vi "Graphics-Create Gradient.vi"(0 "intensity graph":refnum<vi>, 5 "Color 1":u32(colorbox)=16777216, 7 "Color 2":u32(colorbox)=16777215, 9 "Fraction":dbl, 11 "error in (no error)":errorcluster, 12 "Direction":T1(ring), 13 "Frame Color":u32(colorbox)=16777216) -> (15 "error out":errorcluster)   [LabVIEW 2020]
uses:
  Math VIs/LinSpace (x0-dx-npts).vi
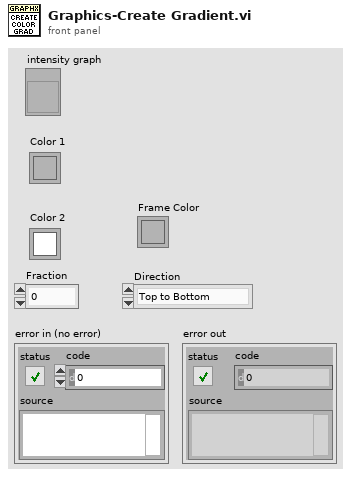
[diagram p1: front panel]
types:
  T1 = enum16{"Top to Bottom", "Bottom to Top", "Left to Right", "Right to Left"}
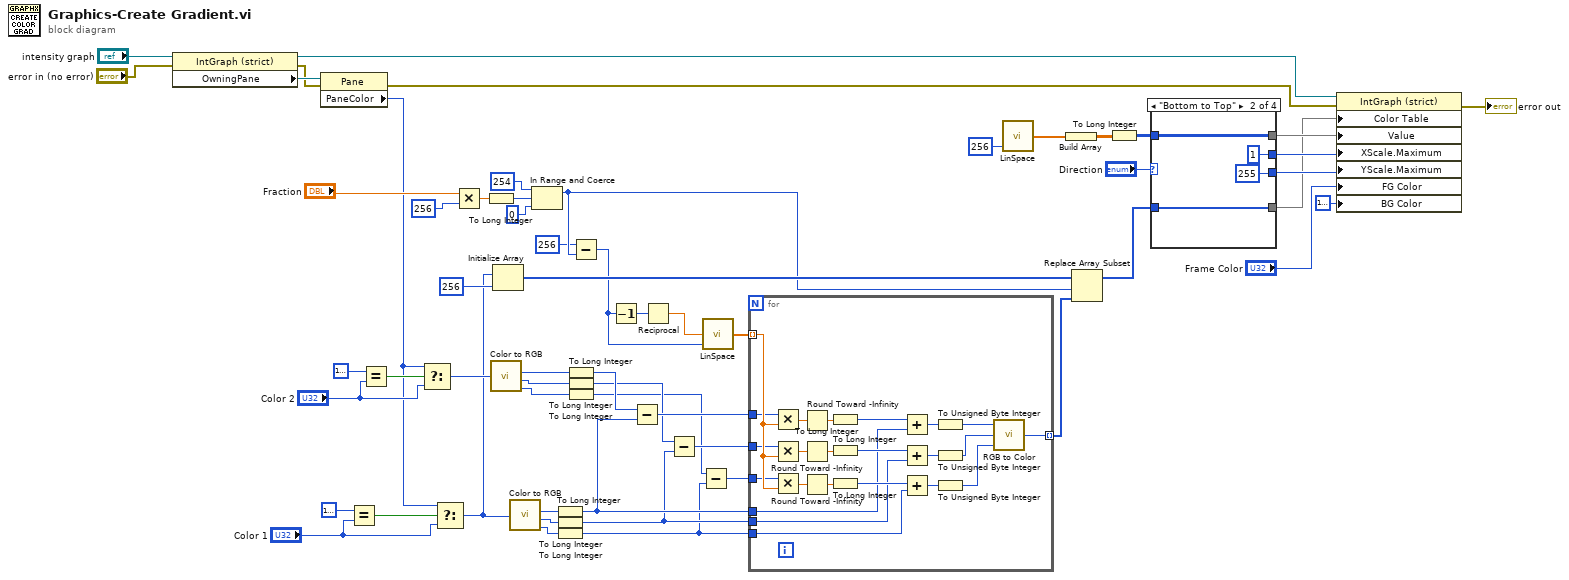
[diagram p0: block diagram]
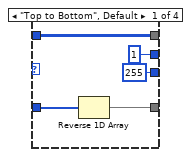
[diagram p2: hidden frame]
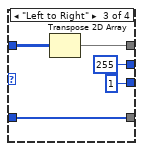
[diagram p3: hidden frame]
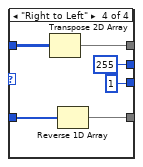
[diagram p4: hidden frame]
diagram:
  n1 = property class="IntGraph (strict)"(reference="intensity graph", error in="error in (no error)") -> (reference out=w11:refnum<vi>, error out=w12:errorcluster, "OwningPane"=w14:refnum<vi>)
  n2 = property class="Pane"(reference=w14, error in=w12) -> (error out=w10:errorcluster, "PaneColor"=w1:u32)  [unwired: 1 out]
  n3 = Equal?(x=u32 16777216, y="Color 1") -> (x = y?=w4:bool)
  n4 = Equal?(x=u32 16777216, y="Color 2") -> (x = y?=w8:bool)
  n5 = Select(t=w1, s=w8, f="Color 2") -> (s? t:f=w6:u32)
  n6 = Select(t=w1, s=w4, f="Color 1") -> (s? t:f=w2:u32)
  n7 = Multiply(x="Fraction", y=256 ("dimension size")) -> (x*y=w37:dbl)
  n8 = To Long Integer(number=w37) -> (32bit integer=w34:i32)
  n9 = call <vilib>:"Color to RGB.vi"("Color"=w6) -> ("R"=w55:u8, "G"=w53:u8, "B"=w52:u8)  [unwired: 1 out]
  n10 = Initialize Array(w2, 256 ("dimension size")) -> (w33:u32[])
  n11 = call <vilib>:"Color to RGB.vi"("Color"=w2) -> ("R"=w54:u8, "G"=w41:u8, "B"=w51:u8)  [unwired: 1 out]
  n12 = In Range and Coerce(upper limit=254, x=w34, lower limit=0) -> (coerced(x)=w29:i32)  [unwired: 1 out]
  n13 = To Long Integer(number=w54) -> (32bit integer=w44:i32)
  n14 = To Long Integer(number=w41) -> (32bit integer=w43:i32)
  n15 = To Long Integer(number=w51) -> (32bit integer=w42:i32)
  n16 = To Long Integer(number=w55) -> (32bit integer=w47:i32)
  n17 = To Long Integer(number=w53) -> (32bit integer=w46:i32)
  n18 = To Long Integer(number=w52) -> (32bit integer=w45:i32)
  n19 = Subtract(x=256, y=w29) -> (x-y=w27:i32)
  n20 = Decrement(x=w27) -> (x-1=w26:i32)
  n21 = Subtract(x=w47, y=w44) -> (x-y=w50:i32)
  n22 = Reciprocal(x=w26) -> (1/x=w25:dbl)
  n23 = Subtract(x=w46, y=w43) -> (x-y=w49:i32)
  n24 = Subtract(x=w45, y=w42) -> (x-y=w48:i32)
  n25 = call-poly "LinSpace.vi"("npts"=w27, "dx"=w25) -> ("Array"=w36:dbl[])  [unwired: 2 in, 1 out]
  n26 = for {
    tunnel: w36 -> [w75] mode=indexing
    tunnel: [w72] -> w32 mode=indexing
    tunnel: w44 -> [w67]
    tunnel: w43 -> [w66]
    tunnel: w42 -> [w65]
    tunnel: w50 -> [w70]
    tunnel: w49 -> [w69]
    tunnel: w48 -> [w68]
    n27 = Multiply(x=w70, y=w75) -> (x*y=w80:dbl)
    n28 = Multiply(x=w69, y=w75) -> (x*y=w78:dbl)
    n29 = Multiply(x=w68, y=w75) -> (x*y=w76:dbl)
    n30 = Round Toward -Infinity(1:w80) -> (0:w81:dbl)
    n31 = Round Toward -Infinity(1:w78) -> (0:w79:dbl)
    n32 = Round Toward -Infinity(1:w76) -> (0:w77:dbl)
    n33 = To Long Integer(number=w81) -> (32bit integer=w71:i32)
    n34 = To Long Integer(number=w79) -> (32bit integer=w74:i32)
    n35 = To Long Integer(number=w77) -> (32bit integer=w73:i32)
    n36 = Add(x=w71, y=w67) -> (x+y=w64:i32)
    n37 = Add(x=w74, y=w66) -> (x+y=w63:i32)
    n38 = Add(x=w73, y=w65) -> (x+y=w62:i32)
    n39 = To Unsigned Byte Integer(number=w64) -> (unsigned 8bit integer=w61:u8)
    n40 = To Unsigned Byte Integer(number=w63) -> (unsigned 8bit integer=w60:u8)
    n41 = To Unsigned Byte Integer(number=w62) -> (unsigned 8bit integer=w59:u8)
    n42 = call <vilib>:"RGB to Color.vi"("B"=w59, "G"=w60, "R"=w61) -> ("Color"=w72:u32)
  }
  n43 = call-poly "LinSpace.vi"("npts"=256) -> ("Array"=w56:dbl[])  [unwired: 3 in, 1 out]
  n44 = Build Array(w56) -> (w57:dbl[][])
  n45 = Replace Array Subset(array=w33, new element=w32, index=w29) -> (w19:u32[])
  n46 = To Long Integer(number=w57) -> (32bit integer=w20:i32[][])
  n47 = case shown="\"Bottom to Top\"" "Direction" {
    tunnel: [1 1 255 255] -> w23
    tunnel: [255 255 1 1] -> w22
    tunnel: [w84 w90 w92 w98] -> w21
    tunnel: w20 -> [w84 w90 w93 w99]
    tunnel: w19 -> [w83 w87 w91 w97]
    tunnel: [w82 w87 w91 w96] -> w18
    frame "Top to Bottom", Default {
      n48 = Reverse 1D Array(array=w83) -> (reversed array=w82:u32[])
    }
    frame "Bottom to Top" {
    }
    frame "Left to Right" {
      n49 = Transpose 2D Array(2D array=w93) -> (transposed array=w92:i32[][])
    }
    frame "Right to Left" {
      n50 = Transpose 2D Array(2D array=w99) -> (transposed array=w98:i32[][])
      n51 = Reverse 1D Array(array=w97) -> (reversed array=w96:u32[])
    }
  }
  n52 = property on="Property Node" class="IntGraph (strict)"(reference=w11, error in=w10, "Color Table"=w18, "Value"=w21, "XScale.Maximum"=w23, "YScale.Maximum"=w22, "FG Color"="Frame Color", "BG Color"=u32 16777216) -> (error out=→"error out":errorcluster)  [unwired: 1 out]
